vi "Mod_OFDM_Config_OFDM_Symbol.vi"(0 "Configuration in":variant=variant("Attribute Names"=variant(cluster{"Data Source Pool":string, "Modulator Source Pool":string, "OFDM SYMBOL POOL":string, "Symbol Table":string, "Sub Carrier Selection":string, "OFDM Frame":string, "FRAME Table":string, "Pulse Shaping":string} {"Data Source Pool"="Data Source ", "Modulator Source Pool"="Modulator Source Pool ", "OFDM SYMBOL POOL"="OFDM SYMBOL POOL", "Symbol Table"="Symbol Table", "Sub Carrier Selection"="Sub Carrier Selection", "OFDM Frame"="OFDM Frame", "FRAME Table"="FRAME Table", "Pulse Shaping"="Pulse Shaping"}), "Data Source "=variant(cluster{"mode (PN)":enum16{"PN", "pattern", "user"}, "PN sequence order (9)":i32, "Invert Output Bits":enum16{"No", "Yes"}, "Register Initial State":u32, "User base bit pattern":i8[], "base bit pattern (00001111)":enum16{"0", "1", "01", "0011", "00001111"}, "Reset to Initial State":enum16{"Every OFDM Frame", "Every OFDM Symbol", "Every Sub Carrier"}}[] [{"mode (PN)"=enum."PN", "PN sequence order (9)"=9, "Invert Output Bits"=enum."No", "Register Initial State"=3602873842, "User base bit pattern"=[], "base bit pattern (00001111)"=enum."00001111", "Reset to Initial State"=enum."Every OFDM Frame"}, {"mode (PN)"=enum."PN", "PN sequence order (9)"=9, "Invert Output Bits"=enum."No", "Register Initial State"=3602873842, "User base bit pattern"=[], "base bit pattern (00001111)"=enum."00001111", "Reset to Initial State"=enum."Every OFDM Frame"}, {"mode (PN)"=enum."PN", "PN sequence order (9)"=9, "Invert Output Bits"=enum."No", "Register Initial State"=3602873842, "User base bit pattern"=[], "base bit pattern (00001111)"=enum."00001111", "Reset to Initial State"=enum."Every OFDM Frame"}, {"mode (PN)"=enum."PN", "PN sequence order (9)"=9, "Invert Output Bits"=enum."No", "Register Initial State"=3602873842, "User base bit pattern"=[], "base bit pattern (00001111)"=enum."00001111", "Reset to Initial State"=enum."Every OFDM Frame"}]), "FRAME Table"=variant(string[][] []), "Modulator Source Pool "=variant(cluster{"M-QAM":enum16{"4", "16", "64", "256"}, "M-PSK":enum16{"2", "4", "8", "16", "32", "64", "128", "256"}, "Type of Modulation":enum16{"PSK", "QAM"}, "PSK":cluster{"differential PSK":enum16{"disable", "enable"}, "PSK type":enum16{"normal", "shifted", "offset"}}}[] [{"M-QAM"=enum."4", "M-PSK"=enum."2", "Type of Modulation"=enum."PSK", "PSK"={"differential PSK"=enum."disable", "PSK type"=enum."normal"}}, {"M-QAM"=enum."4", "M-PSK"=enum."2", "Type of Modulation"=enum."PSK", "PSK"={"differential PSK"=enum."disable", "PSK type"=enum."normal"}}, {"M-QAM"=enum."4", "M-PSK"=enum."2", "Type of Modulation"=enum."PSK", "PSK"={"differential PSK"=enum."disable", "PSK type"=enum."normal"}}, {"M-QAM"=enum."4", "M-PSK"=enum."2", "Type of Modulation"=enum."PSK", "PSK"={"differential PSK"=enum."disable", "PSK type"=enum."normal"}}]), "OFDM Frame"=variant(cluster{"Symbol Name":string, "# of Symbols":i32}[] []), "OFDM SYMBOL POOL"=variant(string[] []), "Pulse Shaping"=variant(cluster{"System Filter":cluster{"TX Filter":enum16{"none", "Raised Cosine", "Root Raised Cos"}, "Alpha":dbl, "filter length":i32}, "Modulation system parameters":cluster{"samples per symbol (16)":i32}, "symbol rate (Hz)":dbl} {"System Filter"={"TX Filter"=enum."Raised Cosine", "Alpha"=0.5, "filter length"=8}, "Modulation system parameters"={"samples per symbol (16)"=16}, "symbol rate (Hz)"=100000.0}), "Sub Carrier Selection"=variant(cluster{"Sub Carrier Selection":cluster{"Sub Carrier":bool, "Data Source":u16, "Modulator":u16}[], "OFDM Parameters":cluster{"# of Sub Carrier":i32, "Length Of Cylic Prefix":i32}} {"Sub Carrier Selection"=[{"Sub Carrier"=TRUE, "Data Source"=0, "Modulator"=0}, {"Sub Carrier"=TRUE, "Data Source"=0, "Modulator"=0}, {"Sub Carrier"=TRUE, "Data Source"=0, "Modulator"=0}, {"Sub Carrier"=TRUE, "Data Source"=0, "Modulator"=0}, {"Sub Carrier"=TRUE, "Data Source"=0, "Modulator"=0}, {"Sub Carrier"=TRUE, "Data Source"=0, "Modulator"=0}], "OFDM Parameters"={"# of Sub Carrier"=64, "Length Of Cylic Prefix"=16}}), "Symbol Table"=variant(string[][] [])), 1 "Data Source Name":string[](array[string])=["Data Source 0", "Data Source 1", "Data Source 2", "Data Source 3"], 5 "OFDM PARAMETERS":T5={"# of Sub Carrier"=64, "Length Of Cylic Prefix"=16}, 7 "DATA Source Pool":T4=[{"mode (PN)"=enum."PN", "PN sequence order (9)"=9, "Invert Output Bits"=enum."No", "Register Initial State "=3602873842, "User base bit pattern"=[], "base bit pattern (00001111)"=enum."00001111", "Reset to Initial State"=enum."Every OFDM Frame"}, {"mode (PN)"=enum."PN", "PN sequence order (9)"=9, "Invert Output Bits"=enum."No", "Register Initial State "=3602873842, "User base bit pattern"=[], "base bit pattern (00001111)"=enum."00001111", "Reset to Initial State"=enum."Every OFDM Frame"}, {"mode (PN)"=enum."PN", "PN sequence order (9)"=9, "Invert Output Bits"=enum."No", "Register Initial State "=3602873842, "User base bit pattern"=[], "base bit pattern (00001111)"=enum."00001111", "Reset to Initial State"=enum."Every OFDM Frame"}, {"mode (PN)"=enum."PN", "PN sequence order (9)"=9, "Invert Output Bits"=enum."No", "Register Initial State "=3602873842, "User base bit pattern"=[], "base bit pattern (00001111)"=enum."00001111", "Reset to Initial State"=enum."Every OFDM Frame"}] {"Register Initial State" format="%08x"}, 9 "Modulator Pool":T3=[{"M-QAM"=enum."4", "M-PSK"=enum."2", "Type of Modulation"=enum."PSK", " PSK"={"differential PSK"=enum."disable", "PSK type"=enum."normal"}}, {"M-QAM"=enum."4", "M-PSK"=enum."2", "Type of Modulation"=enum."PSK", " PSK"={"differential PSK"=enum."disable", "PSK type"=enum."normal"}}, {"M-QAM"=enum."4", "M-PSK"=enum."2", "Type of Modulation"=enum."PSK", " PSK"={"differential PSK"=enum."disable", "PSK type"=enum."normal"}}, {"M-QAM"=enum."4", "M-PSK"=enum."2", "Type of Modulation"=enum."PSK", " PSK"={"differential PSK"=enum."disable", "PSK type"=enum."normal"}}], 11 "error in":errorcluster, 14 "Modulator Source Name":string[](array[string])=["Modulator 0", "Modulator 1", "Modulator 2", "Modulator 3"]) -> (4 "Configuration out":variant=variant("Attribute Names"=variant(cluster{"Data Source Pool":string, "Modulator Source Pool":string, "OFDM SYMBOL POOL":string, "Symbol Table":string, "Sub Carrier Selection":string, "OFDM Frame":string, "FRAME Table":string, "Pulse Shaping":string} {"Data Source Pool"="Data Source ", "Modulator Source Pool"="Modulator Source Pool ", "OFDM SYMBOL POOL"="OFDM SYMBOL POOL", "Symbol Table"="Symbol Table", "Sub Carrier Selection"="Sub Carrier Selection", "OFDM Frame"="OFDM Frame", "FRAME Table"="FRAME Table", "Pulse Shaping"="Pulse Shaping"}), "Data Source "=variant(cluster{"mode (PN)":enum16{"PN", "pattern", "user"}, "PN sequence order (9)":i32, "Invert Output Bits":enum16{"No", "Yes"}, "Register Initial State":u32, "User base bit pattern":i8[], "base bit pattern (00001111)":enum16{"0", "1", "01", "0011", "00001111"}, "Reset to Initial State":enum16{"Every OFDM Frame", "Every OFDM Symbol", "Every Sub Carrier"}}[] [{"mode (PN)"=enum."PN", "PN sequence order (9)"=9, "Invert Output Bits"=enum."No", "Register Initial State"=3602873842, "User base bit pattern"=[], "base bit pattern (00001111)"=enum."00001111", "Reset to Initial State"=enum."Every OFDM Frame"}, {"mode (PN)"=enum."PN", "PN sequence order (9)"=9, "Invert Output Bits"=enum."No", "Register Initial State"=3602873842, "User base bit pattern"=[], "base bit pattern (00001111)"=enum."00001111", "Reset to Initial State"=enum."Every OFDM Frame"}, {"mode (PN)"=enum."PN", "PN sequence order (9)"=9, "Invert Output Bits"=enum."No", "Register Initial State"=3602873842, "User base bit pattern"=[], "base bit pattern (00001111)"=enum."00001111", "Reset to Initial State"=enum."Every OFDM Frame"}, {"mode (PN)"=enum."PN", "PN sequence order (9)"=9, "Invert Output Bits"=enum."No", "Register Initial State"=3602873842, "User base bit pattern"=[], "base bit pattern (00001111)"=enum."00001111", "Reset to Initial State"=enum."Every OFDM Frame"}]), "FRAME Table"=variant(string[][] []), "Modulator Source Pool "=variant(cluster{"M-QAM":enum16{"4", "16", "64", "256"}, "M-PSK":enum16{"2", "4", "8", "16", "32", "64", "128", "256"}, "Type of Modulation":enum16{"PSK", "QAM"}, "PSK":cluster{"differential PSK":enum16{"disable", "enable"}, "PSK type":enum16{"normal", "shifted", "offset"}}}[] [{"M-QAM"=enum."4", "M-PSK"=enum."2", "Type of Modulation"=enum."PSK", "PSK"={"differential PSK"=enum."disable", "PSK type"=enum."normal"}}, {"M-QAM"=enum."4", "M-PSK"=enum."2", "Type of Modulation"=enum."PSK", "PSK"={"differential PSK"=enum."disable", "PSK type"=enum."normal"}}, {"M-QAM"=enum."4", "M-PSK"=enum."2", "Type of Modulation"=enum."PSK", "PSK"={"differential PSK"=enum."disable", "PSK type"=enum."normal"}}, {"M-QAM"=enum."4", "M-PSK"=enum."2", "Type of Modulation"=enum."PSK", "PSK"={"differential PSK"=enum."disable", "PSK type"=enum."normal"}}]), "OFDM Frame"=variant(cluster{"Symbol Name":string, "# of Symbols":i32}[] []), "OFDM SYMBOL POOL"=variant(string[] []), "Pulse Shaping"=variant(cluster{"System Filter":cluster{"TX Filter":enum16{"none", "Raised Cosine", "Root Raised Cos"}, "Alpha":dbl, "filter length":i32}, "Modulation system parameters":cluster{"samples per symbol (16)":i32}, "symbol rate (Hz)":dbl} {"System Filter"={"TX Filter"=enum."Raised Cosine", "Alpha"=0.5, "filter length"=8}, "Modulation system parameters"={"samples per symbol (16)"=16}, "symbol rate (Hz)"=100000.0}), "Sub Carrier Selection"=variant(cluster{"Sub Carrier Selection":cluster{"Sub Carrier":bool, "Data Source":u16, "Modulator":u16}[], "OFDM Parameters":cluster{"# of Sub Carrier":i32, "Length Of Cylic Prefix":i32}} {"Sub Carrier Selection"=[{"Sub Carrier"=TRUE, "Data Source"=0, "Modulator"=0}, {"Sub Carrier"=TRUE, "Data Source"=0, "Modulator"=0}, {"Sub Carrier"=TRUE, "Data Source"=0, "Modulator"=0}, {"Sub Carrier"=TRUE, "Data Source"=0, "Modulator"=0}, {"Sub Carrier"=TRUE, "Data Source"=0, "Modulator"=0}, {"Sub Carrier"=TRUE, "Data Source"=0, "Modulator"=0}], "OFDM Parameters"={"# of Sub Carrier"=64, "Length Of Cylic Prefix"=16}}), "Symbol Table"=variant(string[][] [])), 15 "error out":errorcluster)   [LabVIEW 2010]
uses:
  Controls(Type_DEf)/Pool of Data Source Control.ctl
  Controls(Type_DEf)/Pool of Modulator Control.ctl
  Polymorphic_Sub_VI's/MOD_OFDM_Get_Attr.vi
  Polymorphic_Sub_VI's/Mod_OFDM_Set_Ofdm_Symbol.vi
  Polymorphic_Sub_VI's/Mod_OFDM_Set_Ofdm_Symbol_Pool.vi
panel:
  out "Symbol Table":string[][](table)=[["-32", "OFF", "0", "1"], ["-31", "OFF", "0", "1"], ["-30", "OFF", "0", "1"], ["-29", "OFF", "0", "1"], ["-28", "OFF", "0", "1"], ["-27", "OFF", "0", "1"], ["-26", "OFF", "0", "1"], ["-25", " ON", "0", "1"], ["-24", " ON", "0", "1"], ["-23", " ON", "0", "1"], ["-22", " ON", "0", "1"], ["-21", " ON", "1", "1"], ["-20", " ON", "0", "1"], ["-19", " ON", "0", "1"], ["-18", " ON", "0", "1"], ["-17", " ON", "0", "1"], ["-16", " ON", "0", "1"], ["-15", " ON", "0", "1"], ["-14", " ON", "0", "1"], ["-13", " ON", "0", "1"], ["-12", " ON", "0", "1"], ["-11", " ON", "0", "1"], ["-10", " ON", "0", "1"], ["-9", " ON", "0", "1"], ["-8", " ON", "0", "1"], ["-7", " ON", "1", "1"], ["-6", " ON", "0", "1"], ["-5", " ON", "0", "1"], ["-4", " ON", "0", "1"], ["-3", " ON", "0", "1"], ["-2", " ON", "0", "1"], ["-1", " ON", "0", "1"], ["0", "OFF", "0", "1"], ["+1", " ON", "0", "1"], ["+2", " ON", "0", "1"], ["+3", " ON", "0", "1"], ["+4", " ON", "0", "1"], ["+5", " ON", "0", "1"], ["+6", " ON", "0", "1"], ["+7", " ON", "1", "1"], ["+8", " ON", "0", "1"], ["+9", " ON", "0", "1"], ["+10", " ON", "0", "1"], ["+11", " ON", "0", "1"], ["+12", " ON", "0", "1"], ["+13", " ON", "0", "1"], ["+14", " ON", "0", "1"], ["+15", " ON", "0", "1"], ["+16", " ON", "0", "1"], ["+17", " ON", "0", "1"], ["+18", " ON", "0", "1"], ["+19", " ON", "0", "1"], ["+20", " ON", "0", "1"], ["+21", " ON", "2", "1"], ["+22", " ON", "0", "1"], ["+23", " ON", "0", "1"], ["+24", " ON", "0", "1"], ["+25", " ON", "0", "1"], ["+26", " ON", "0", "1"], ["+27", "OFF", "0", "1"], ["+28", "OFF", "0", "1"], ["+29", "OFF", "0", "1"], ["+30", "OFF", "0", "1"], ["+31", "OFF", "0", "1"]]
  out "Data Source":T1={"mode (PN)"=enum."PN", "PN sequence order (9)"=9, "Invert Output Bits"=enum."No", "Register Initial State"=3602873842, "User base bit pattern"=[], "base bit pattern"=enum."00001111", "Reset to Initial State"=enum."Every OFDM Frame"} {"Register Initial State" format="%08x"}
  out "Modulator":T2
  in  "Symbol Pool":u16(ring) items=["IEEE 802.11a First Symbol of Frame", "IEEE 802.11a Frame (BPSK)", "IEEE 802.11a Frame (QPSK)", "IEEE 802.11a Frame (16QAM)", "IEEE 802.11a Frame (64QAM)"]
  in  "Current Symbol Name":string
  in  "APPLY SETTINGS":bool
  in  "Cancel Operation":bool
  in  "OK":bool
  in  "Modulator":i32(ring) items=["Modulator 0", "Modulator 1", "Modulator 2", "Modulator 3"]
  in  "Data Source":i32(ring) items=["Data Source 0", "Data Source 1", "Data Source 2", "Data Source 3"]
  in  "Sub Carrier":bool=TRUE
  in  "RANGE/SINGLE":T6(tab)
  in  "To":i32=31 min=-32 max=31 step=1
  in  "From":i32=-32 min=-32 max=31 step=1
  in  "Single Subcarrier":i32=15 min=-32 max=31 step=1
  # "Sub\nCarrier"
  # "Data \nSource"
  # "Modulator\nSource"
  # "State"
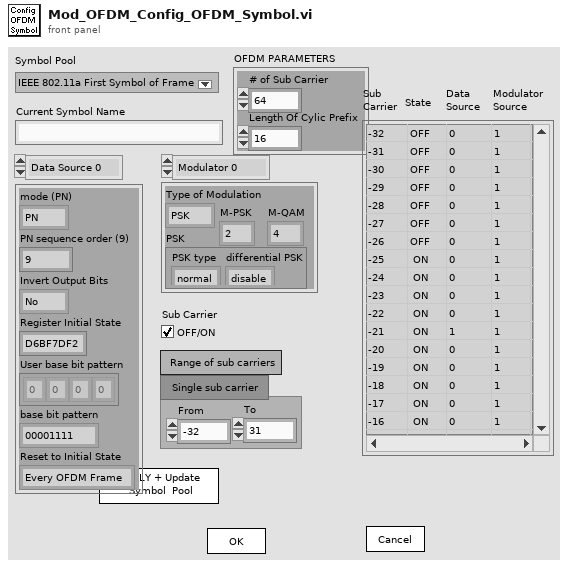
[diagram p1: front panel]
types:
  T1 = cluster{"mode (PN)":enum16{"PN", "pattern", "user"}, "PN sequence order (9)":i32, "Invert Output Bits":enum16{"No", "Yes"}, "Register Initial State":u32, "User base bit pattern":i8[], "base bit pattern":enum16{"0", "1", "01", "0011", "00001111"}, "Reset to Initial State":enum16{"Every OFDM Frame", "Every OFDM Symbol", "Every Sub Carrier"}}
  T2 = cluster{"M-QAM":enum16{"4", "16", "64", "256", "1024"}, "M-PSK":enum16{"2", "4", "8", "16", "32", "64", "128", "256"}, "Type of Modulation":enum16{"PSK", "QAM"}, "PSK":cluster{"differential PSK":enum16{"disable", "enable"}, "PSK type":enum16{"normal", "shifted", "offset"}}}
  T3 = typedef "Pool of Modulator Control.ctl" = cluster{"M-QAM":enum16{"4", "16", "64", "256"}, "M-PSK":enum16{"2", "4", "8", "16", "32", "64", "128", "256"}, "Type of Modulation":enum16{"PSK", "QAM"}, " PSK":cluster{"differential PSK":enum16{"disable", "enable"}, "PSK type":enum16{"normal", "shifted", "offset"}}}[]
  T4 = typedef "Pool of Data Source Control.ctl" = cluster{"mode (PN)":enum16{"PN", "pattern", "user"}, "PN sequence order (9)":i32, "Invert Output Bits":enum16{"No", "Yes"}, "Register Initial State ":u32, "User base bit pattern":i8[], "base bit pattern (00001111)":enum16{"0", "1", "01", "0011", "00001111"}, "Reset to Initial State":enum16{"Every OFDM Frame", "Every OFDM Symbol", "Every Sub Carrier"}}[]
  T5 = cluster{"# of Sub Carrier":i32, "Length Of Cylic Prefix":i32}
  T6 = enum32{" Range of sub carriers", "Single sub carrier   "}
  T7 = cluster{"Minimum":i32, "Maximum":i32, "Increment":i32}
  T8 = cluster{"M-QAM":enum16{"4", "16", "64", "256"}, "M-PSK":enum16{"2", "4", "8", "16", "32", "64", "128", "256"}, "Type of Modulation":enum16{"PSK", "QAM"}, " PSK":cluster{"differential PSK":enum16{"disable", "enable"}, "PSK type":enum16{"normal", "shifted", "offset"}}}
  T9 = cluster{"mode (PN)":enum16{"PN", "pattern", "user"}, "PN sequence order (9)":i32, "Invert Output Bits":enum16{"No", "Yes"}, "Register Initial State ":u32, "User base bit pattern":i8[], "base bit pattern (00001111)":enum16{"0", "1", "01", "0011", "00001111"}, "Reset to Initial State":enum16{"Every OFDM Frame", "Every OFDM Symbol", "Every Sub Carrier"}}
  T10 = cluster{"RANGE/SINGLE":enum32{" Range of sub carriers", "Single sub carrier   "}, "From ":i32, "To ":i32, "Single Subcarrier":i32, "Modulator":i32, "Data Source":i32, "Sub Carrier":bool}
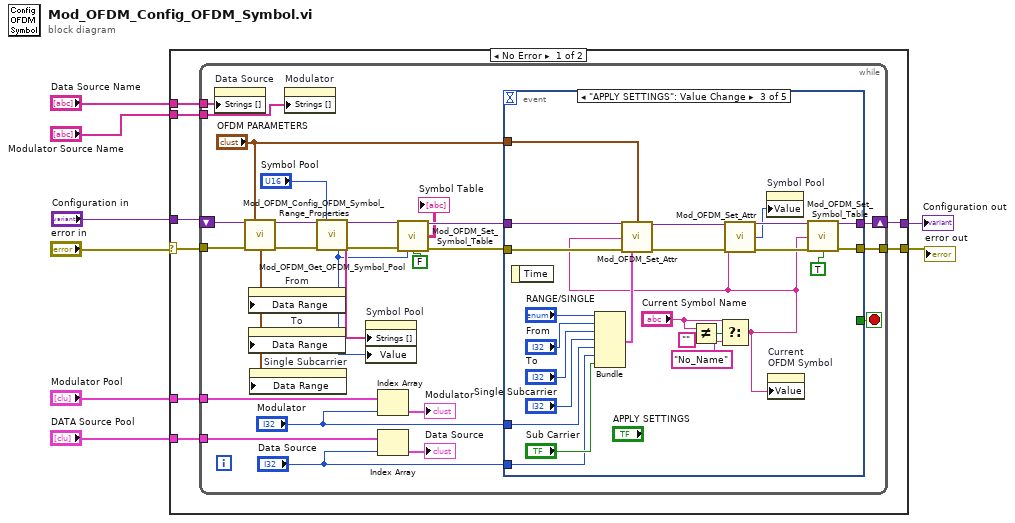
[diagram p0: block diagram]
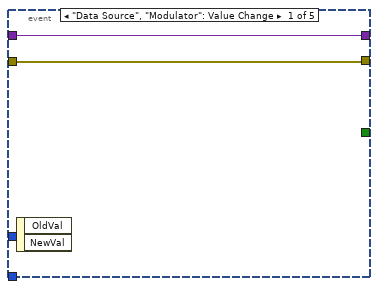
[diagram p2: hidden frame]
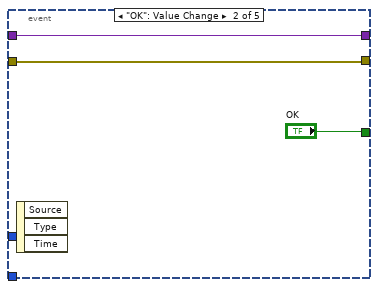
[diagram p3: hidden frame]
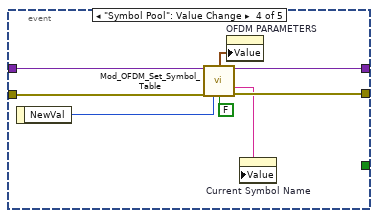
[diagram p4: hidden frame]
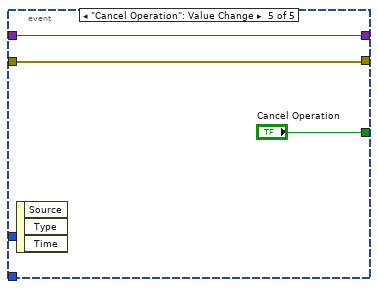
[diagram p5: hidden frame]
diagram:
  n1 = case shown="No Error" "error in" {
    selector: "error in" -> [w10 w82]
    tunnel: [w16 _] -> w8
    tunnel: "Configuration in" -> [w15 _]
    tunnel: "Data Source Name" -> [w14 _]
    tunnel: "Modulator Source Name" -> [w13 _]
    tunnel: "Modulator Pool" -> [w12 _]
    tunnel: "DATA Source Pool" -> [w11 _]
    tunnel: [w9 w82] -> w1
    frame No Error {
      n2 = while {
        shift-right: [w39] -> w16
        shift-left: w15 -> [w27]
        tunnel: w14 -> [w35]
        tunnel: w13 -> [w40]
        tunnel: w12 -> [w38]
        tunnel: w11 -> [w37]
        tunnel: w10 -> [w34]
        tunnel: [w36] -> w9
        stop <- w41 stop-if-true
        n3 = property on="Data Source" class="Ring (strict)"("Strings []"=w35) -> ()  [unwired: 2 in, 2 out]
        n4 = call "Mod_OFDM_Config_OFDM_Symbol_Range_Properties.vi"("OFDM PARAMETERS"="OFDM PARAMETERS", "error in"=w34) -> ("Data Range"=w32:T7, "error out"=w26:errorcluster)  [unwired: 12 in]
        n5 = property on="From" class="DigNum (strict)"("Data Range"=w32) -> ()  [unwired: 2 in, 2 out]
        n6 = property on="To" class="DigNum (strict)"("Data Range"=w32) -> ()  [unwired: 2 in, 2 out]
        n7 = property on="Single Subcarrier" class="DigNum (strict)"("Data Range"=w32) -> ()  [unwired: 2 in, 2 out]
        n8 = property on="Modulator" class="Ring (strict)"("Strings []"=w40) -> ()  [unwired: 2 in, 2 out]
        n9 = call-poly "Mod_OFDM_Get_OFDM_Symbol_Pool.vi"("Configuration in"=w27, "Symbol Pool"="Symbol Pool", "error in"=w26) -> ("Configuration out"=w25:variant, 8:"Symbol Pool"=w20:string[], 14:"Symbol Pool"=w19:u16, "error out"=w24:errorcluster)  [unwired: 7 in, 2 out]
        n10 = property on="Symbol Pool" class="Ring (strict)"("Strings []"=w20, "Value"=w19) -> ()  [unwired: 2 in, 2 out]
        n11 = Index Array(array=w38, index="Modulator") -> (element=→"Modulator":T8)
        n12 = Index Array(array=w37, index="Data Source") -> (element=→"Data Source":T9)
        n13 = call "Mod_OFDM_Set_Symbol_Table.vi"("Configuration in"=w25, "error in"=w24, "Symbol Pool"=w19, "Configure/\nRetrieve"=FALSE ("Configure/\nRetrieve")) -> ("Configuration out"=w22:variant, "Symbol Table"=→"Symbol Table":string[][], "error out"=w21:errorcluster)  [unwired: 7 in, 2 out]
        n14 = event shown="[2] \"APPLY SETTINGS \": Value Change" {
          selector: _ -> [_ _ _ _ _]
          dyn-events: _ -> [_ _ _ _ _]
          timeout: _ -> [_ _ _ _ _]
          tunnel: [_ "OK" _ _ "Cancel Operation"] -> w41
          tunnel: [w43 w45 w69 w76 w80] -> w39
          tunnel: w22 -> [w43 w45 w70 w77 w80]
          tunnel: w21 -> [w42 w44 w60 w75 w79]
          tunnel: [w42 w44 w59 w74 w79] -> w36
          tunnel: "OFDM PARAMETERS" -> [_ _ w58 _ _]
          tunnel: "Modulator" -> [_ _ w49 _ _]
          tunnel: "Data Source" -> [_ _ w48 _ _]
          event "OFDM PARAMETERS.# of Sub Carrier", "Data Source", "Modulator": Value Change {
            n15 = event-data() -> ()  [unwired: 1 in, 2 out]
          }
          event "OK": Value Change {
            n16 = event-data() -> ()  [unwired: 1 in, 3 out]
          }
          event "APPLY SETTINGS": Value Change {
            n17 = event-data() -> ()  [unwired: 1 in, 1 out]
            n18 = Bundle("RANGE/SINGLE"="RANGE/SINGLE", "From"="From", "To"="To", "Single Subcarrier"="Single Subcarrier", "Modulator"=w49, "Data Source"=w48, "Sub Carrier"="Sub Carrier") -> (w50:T10)  [unwired: 1 in]
            n19 = Not Equal?(x="Current Symbol Name", y="") -> (x != y?=w62:bool)
            n20 = Select(t="Current Symbol Name", s=w62, f="No_Name") -> (s? t:f=w47:string)
            n21 = call-poly "Mod_OFDM_Set_Attr.vi"("Configuration out"=w70, "OFDM PARAMETERS"=w58, "Current OFDM Symbol"=w47, "error in"=w60, "Configure OFDM\nSymbol Settings"=w50) -> ("Configuration out"=w67:variant, "error out"=w65:errorcluster)  [unwired: 9 in]
            n22 = call-poly "Mod_OFDM_Set_Attr.vi"("Configuration out"=w67, "Current OFDM \nSymbol NAME"=w47, "error in"=w65) -> ("Configuration out"=w66:variant, "index of current Symbol"=w57:i32, "error out"=w64:errorcluster)  [unwired: 9 in, 1 out]
            n23 = property on="Symbol Pool" class="Ring (strict)"("Value"=w57) -> ()  [unwired: 2 in, 2 out]
            n24 = property on="Current \nOFDM Symbol" class="Str"("Value"=w47) -> ()  [unwired: 2 in, 2 out]
            n25 = call "Mod_OFDM_Set_Symbol_Table.vi"("Configuration in"=w66, "Current OFDM \nSymbol NAME"=w47, "error in"=w64, "Configure/\nRetrieve"=TRUE ("Configure/\nRetrieve")) -> ("Configuration out"=w69:variant, "error out"=w59:errorcluster)  [unwired: 7 in, 3 out]
          }
          event "Symbol Pool": Value Change {
            n26 = event-data() -> ("NewVal"=w73:u16)  [unwired: 1 in]
            n27 = call "Mod_OFDM_Set_Symbol_Table.vi"("Configuration in"=w77, "error in"=w75, "Symbol Pool"=w73, "Configure/\nRetrieve"=FALSE ("Configure/\nRetrieve")) -> ("OFDM Parameters"=w72:T5, "Configuration out"=w76:variant, "Current OFDM Symbol Name(O/P)"=w71:string, "error out"=w74:errorcluster)  [unwired: 7 in, 1 out]
            n28 = property on="OFDM PARAMETERS" class="Clust (strict)"("Value"=w72) -> ()  [unwired: 2 in, 2 out]
            n29 = property on="Current Symbol Name" class="Str"("Value"=w71) -> ()  [unwired: 2 in, 2 out]
          }
          event "Cancel Operation": Value Change {
            n30 = event-data() -> ()  [unwired: 1 in, 3 out]
          }
        }
      }
    }
    frame Error {
    }
  }
  "Configuration out" <- w8
  "error out" <- w1
